vi "FPGA Image Acquisition (FPGA).vi"() -> ()   [LabVIEW 2013]
doc: "This is the FPGA VI for the 10-Tap 8-Bit Camera with DRAM example. This example demonstrates how to acquire images from a 10-tap, 8-bit, extended configuration, Camera Link camera and transfer the images to the host. This example supports area scan and line scan cameras for both continuous and finite acquisitions.\n\nThis example also demonstrates the use of DRAM as a frame buffer for very high speed acquisitions. Data packing and flow-control are also employed to maximize use of the available DRAM and FIFOs in terms of both memory space and performance.\n\nAdditionally, the example demonstrates the serial server, which allows third-party camera configuration utilities to communicate with the camera using the Camera Link serial interface while this VI is running."
uses:
  Common/CL Signal Mapping.ctl
  Common/CL Configuration.ctl
  <vilib>/Platform/TimedLoop/XDataNode/timing_clust.ctl
  <vilib>/Platform/TimedLoop/XDataNode/nitl_modes.ctl
  <vilib>/Platform/TimedLoop/XDataNode/wakeup.ctl
  <vilib>/rvi/Emulation/niFpgaSctlEmulationGetInTimedLoop.vi
  <vilib>/rvi/Emulation/niFpgaEmulationReportErrorSimple.vi
  <vilib>/rvi/eio/common/nirviEmuTemplateMethod_errors.vi
  <vilib>/rvi/Emulation/niFpgaGetClockAttributes.vi
  <vilib>/rvi/Emulation/niFpgaCriticalErrorInLSC.vi
  Common/CL Data to Pixels/10 Tap 8-Bit.vi
  <vilib>/rvi/interface/RandomDataEmulation/nirviRandomDataFPGAFIFO.vi
  <vilib>/rvi/interface/RandomDataEmulation/niFpgaRandomDataHandleErrors.vi
  <vilib>/rvi/FIFO/Fifo_Resource/nirvififoEmulationWriteFpgaImpl.vi
  <vilib>/rvi/DataTransferAndStorage/Container/Common/niFpgaContainerGetUniqueNameForEmu.vi
  <vilib>/rvi/FIFO/Fifo_Resource/nirvififoEmulationGetNumberOfElementsToReadFpgaImpl.vi
  <vilib>/rvi/FIFO/Fifo_Resource/nirvififoEmulationReadFpgaImpl.vi
  <vilib>/rvi/Emulation/niFpgaProcessEmulError.vi
  <vilib>/Platform/TimedLoop/XDataNode/XDataNode.xnode
  <vilib>/eio/EIONode/EIONode.xnode
  <vilib>/rvi/DataTransferAndStorage/Container/XNode/niFpgaContainer.xnode
  <vilib>/rvi/interface/RandomDataEmulation/nirviRandomDataFpgaReadWriteTemplate.vi
  <vilib>/rvi/FIFO/Fifo_Resource/nirvififoEmulationWrite.vi
  <vilib>/rvi/FIFO/Fifo_Resource/nirvififoEmulationGetNumberOfElementsToRead.vi
  <vilib>/rvi/FIFO/Fifo_Resource/nirvififoEmulationRead.vi
  <vilib>/Platform/TimedLoop/XDataNode/XDNodeRunTimeDep.lvlib
panel:
  in  "CL Config.Configuration":T1=enum."Full"
  in  "CL Config.Signal Mapping":T2=enum."Basler 10-tap"
  in  "CL Config.Line Scan":bool
  in  "CL Config.DVAL Active High":bool=TRUE
  in  "CL Config.LVAL Active High":bool=TRUE
  in  "CL Config.FVAL Active High":bool=TRUE
  in  "CL Config.Spare Active High":bool=TRUE
  in  "Acq Control.Line Scan Height":u32
  in  "Acq Control.Frames To Acq":u32
  in  "Acq Control.Acquire":bool
  in  "Acq Control.Cancel Acq":bool
  in  "Acq Control.Ignore DVAL":bool
  in  "Acq Control.Initialize":bool
  out "Acq Status.Acq In Progress":bool
  out "Acq Status.Clocks Per Line":u32
  out "Acq Status.Frames Acq'd":u32
  out "Acq Status.Lines Per Frame":u32
  out "Acq Status.DMA Write Timeout":bool
  out "Acq Status.Initialized":bool
  in  "UART.Baud Rate":u8
  in  "UART.Transmit":bool
  in  "UART.Tx Data":u8[](array[numeric])=[0, 0, 0, 0, 0, 0, 0, 0, 0, 0] format="%02x"
  in  "UART.Set Baud Rate":bool
  in  "UART.Byte Mode":bool=TRUE
  out "UART.Rx Ready":bool
  out "UART.Break Indicator":bool
  out "UART.Framing Error":bool
  out "UART.Overrun Error":bool
  out "UART.Tx Ready":bool
  out "UART.Rx Data":u8 format="%02x"
  in  "UART.Receive":bool
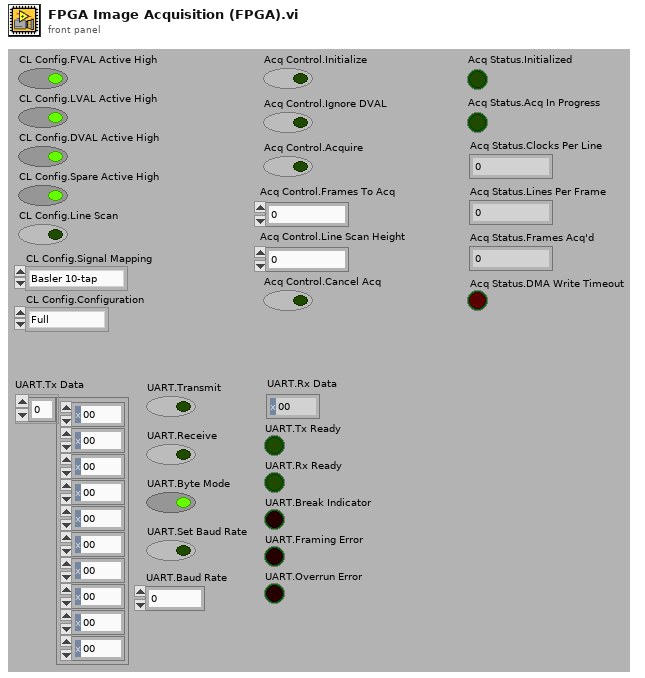
[diagram p1: front panel]
types:
  T1 = typedef "CL Configuration.ctl" = enum8{"Base", "Medium", "Full"}
  T2 = typedef "CL Signal Mapping.ctl" = enum8{"Standard", "Basler 10-tap", "Vosskühler 10-tap"}
  T3 = typedef "XDNodeRunTimeDep.lvlib/timing_clust.ctl" = cluster{"Expected End [f-1]":u64, "Actual End [f-1]":u64, "Finished Late? [f-1]":bool, "Expected End [i-1]":u64, "Actual End [i-1]":u64, "Finished Late? [i-1]":bool, "Expected Start [i]":u64, "Actual Start [i]":u64, "Expected Start [f]":u64, "Actual Start [f]":u64, "Source Name":string, "Structure Name":string, "Period":i64, "Deadline":i64, "Offset":i64, "Start":i64, "Priority":i32, "Timeout":i32, "Mode":T4, "Wakeup Reason":T5, "Error":errorcluster, "Source Type":string, "Secondary Source Type":string, "Global End Time":u64, "Global Start Time":u64, "Frame Duration":u64, "Iteration Duration":u64, "Assigned CPU":i32, "I/O Scan Engine Mode":u32}
  T4 = typedef "XDNodeRunTimeDep.lvlib/nitl_modes.ctl" = enum32{"No Change", "Process missed periods, maintain original phase", "Discard missed periods, maintain original phase", "Process missed periods, ignore original phase", "Discard missed periods, ignore original phase"}
  T5 = typedef "XDNodeRunTimeDep.lvlib/wakeup.ctl" = enum32{"Normal", "Aborted", "Asynchronous wakeup", "Timing source error", "Timed loop error", "Timeout"}
  T6 = cluster{"Enables Valid":bool, "Frame Valid":bool, "Line Valid":bool, "Data Valid":bool}
  T7 = cluster{"Pixel 0":u8, "Pixel 1":u8, "Pixel 2":u8, "Pixel 3":u8, "Pixel 4":u8, "Pixel 5":u8, "Pixel 6":u8, "Pixel 7":u8, "Pixel 8":u8, "Pixel 9":u8}
  T8 = cluster{"Tx Data":u8[], "Transmit":bool, "Receive":bool, "Byte Mode":bool, "Set Baud Rate":bool, "Baud Rate":u8}
  T9 = cluster{"Rx Data":u8, "Turn Off Transmit":bool, "Turn Off Receive":bool, "Turn Off Set Baud Rate":bool, "Tx Ready":bool, "Rx Ready":bool, "Break Indicator":bool, "Framing Error":bool, "Overrun Error":bool}
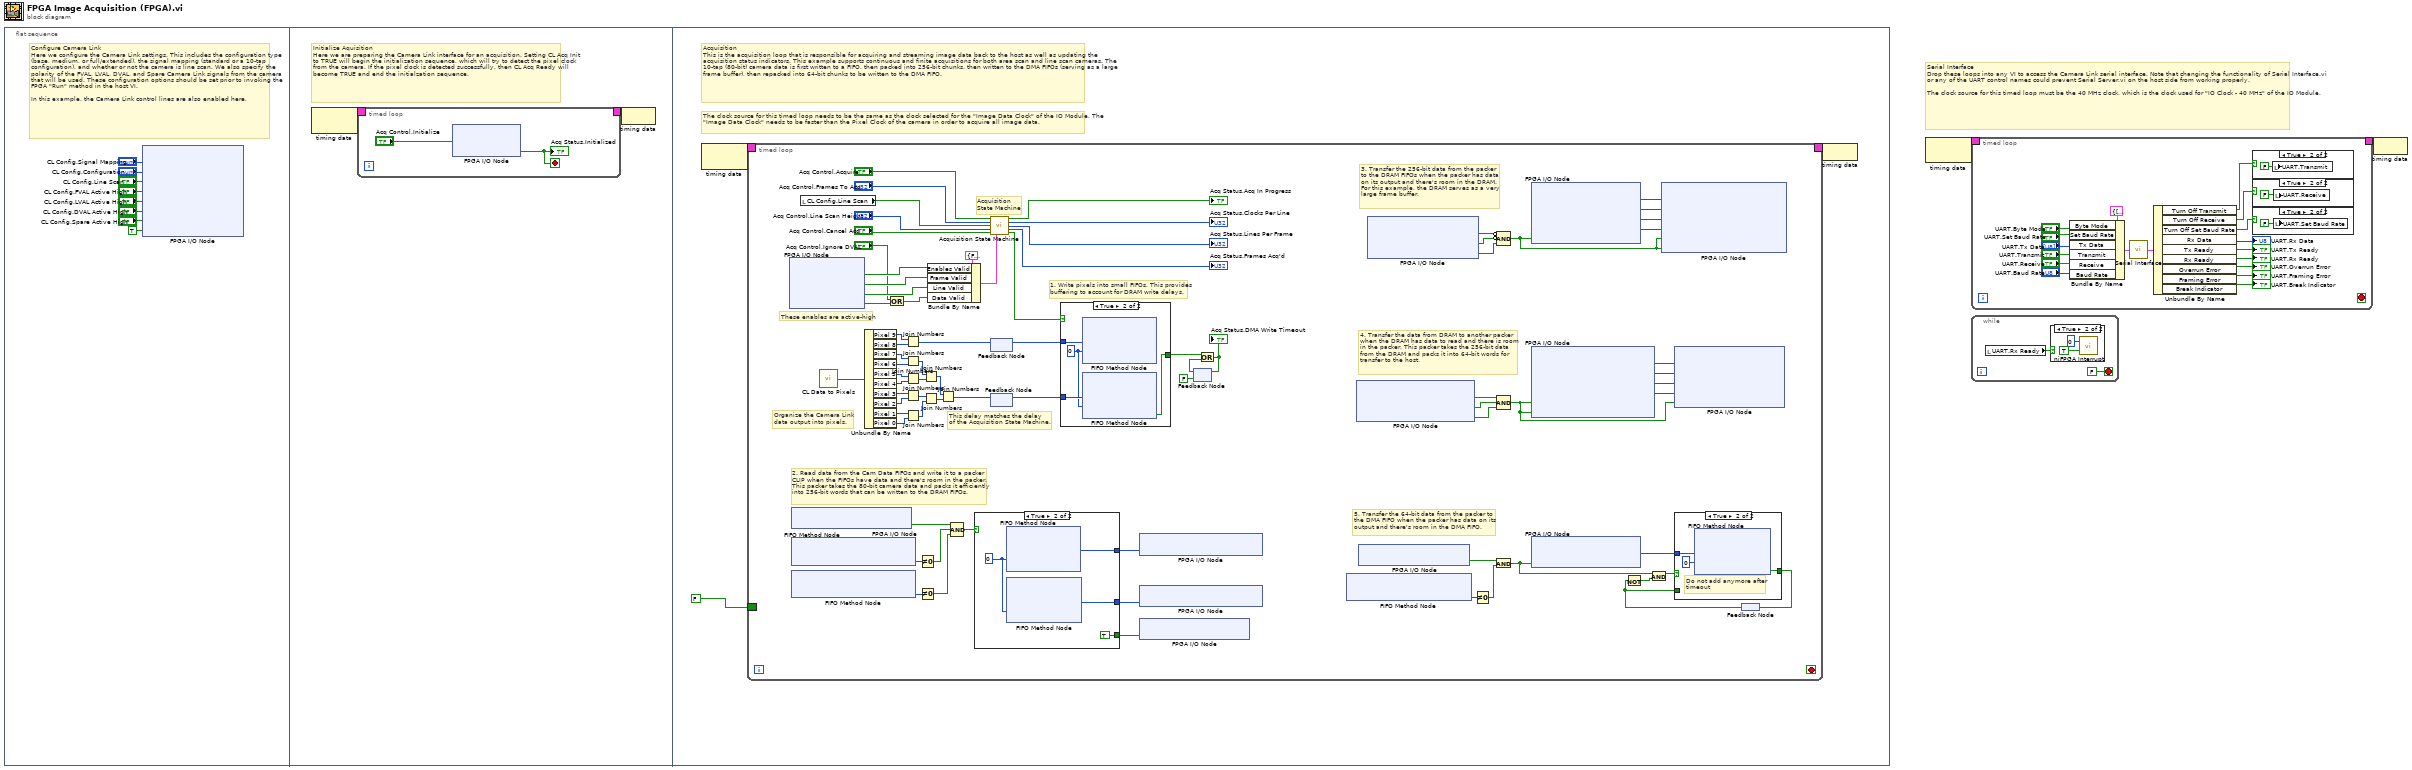
[diagram p0: block diagram]
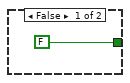
[diagram p8: hidden frame]
diagram:
  # "Serial Interface\nDrop these loops into any VI to access the Camera Link serial interface. Note that changing the functionality of Serial Interface.vi or any of the UART control names could prevent Serial Server.vi on the host side from working properly.\n\nThe clock source for this timed loop must be the 40 MHz clock, which is the clock used for \"IO Clock - 40 MHz\" of the IO Module."
  n1 = flat-sequence {
    frame #0 {
      # "Configure Camera Link\nHere we configure the Camera Link settings. This includes the configuration type (base, medium, or full/extended), the signal mapping (standard or a 10-tap configuration), and whether or not the camera is line scan. We also specify the polarity of the FVAL, LVAL, DVAL, and Spare Camera Link signals from the camera that will be used. These configuration options should be set prior to invoking the FPGA \"Run\" method in the host VI.\n\nIn this example, the Camera Link control lines are also enabled here."
      n2 = xnode "FPGA I/O Node"("CL Set Signal Mapping"="CL Config.Signal Mapping", "CL Set Configuration"="CL Config.Configuration", "CL Set Line Scan"="CL Config.Line Scan", "CL Set FVAL Active High"="CL Config.FVAL Active High", "CL Set LVAL Active High"="CL Config.LVAL Active High", "CL Set DVAL Active High"="CL Config.DVAL Active High", "CL Set Spare Active High"="CL Config.Spare Active High", "CL Control Enable"=TRUE ("IO Module\\CL Control Enable")) -> ()  [unwired: 8 in, 8 out]
    }
    frame #1 {
      # "Initialize Aquisition\nHere we are preparing the Camera Link interface for an acquisition. Setting CL Acq Init to TRUE will begin the initialization sequence, which will try to detect the pixel clock from the camera. If the pixel clock is detected successfully, then CL Acq Ready will become TRUE and end the initialzation sequence."
      n3 = node-c288() -> (w12:T3)  [unwired: 1 out]
      n4 = timed-loop {
        timing: w12 -> [_]
        timing-out: [_] -> w11
        stop <- w13 stop-if-true
        n5 = xnode "FPGA I/O Node"("CL Acq Init"="Acq Control.Initialize") -> ("CL Acq Ready"=w13:bool)  [unwired: 2 in, 2 out]
        "Acq Status.Initialized" <- w13
      }
      n6 = node-c288(w11) -> ()
    }
    frame #2 {
      # "The clock source for this timed loop needs to be the same as the clock selected for the \"Image Data Clock\" of the IO Module. The \"Image Data Clock\" needs to be faster than the Pixel Clock of the camera in order to acquire all image data."
      # "Acquisition\nThis is the acquisition loop that is responsible for acquiring and streaming image data back to the host as well as updating the acquisition status indicators. This example supports continuous and finite acquisitions for both area scan and line scan cameras. The 10-tap (80-bit) camera data is first written to a FIFO, then packed into 256-bit chunks, then written to the DMA FIFOs (serving as a large frame buffer), then repacked into 64-bit chunks to be written to the DMA FIFO."
      n7 = node-c288() -> (w21:T3)  [unwired: 1 in]
      n8 = timed-loop {
        timing: w21 -> [_]
        timing-out: [_] -> w20
        border: FALSE ("Timed Out?") -> [_]
        stop <- _ stop-if-true
        # "3. Transfer the 256-bit data from the packer\nto the DRAM FIFOs when the packer has data\non its output and there's room in the DRAM.\nFor this example, the DRAM serves as a very\nlarge frame buffer."
        # "5. Transfer the 64-bit data from the packer to\nthe DMA FIFO when the packer has data on its\noutput and there's room in the DMA FIFO."
        # "4. Transfer the data from DRAM to another packer\nwhen the DRAM has data to read and there is room\nin the packer. This packer takes the 256-bit data\nfrom the DRAM and packs it into 64-bit words for\ntransfer to the host."
        # "2. Read data from the Cam Data FIFOs and write it to a packer\nCLIP when the FIFOs have data and there's room in the packer.\nThis packer takes the 80-bit camera data and packs it efficiently\ninto 256-bit words that can be written to the DRAM FIFOs."
        # "1. Write pixels into small FIFOs. This provides\nbuffering to account for DRAM write delays."
        # "Organize the Camera Link\ndata output into pixels."
        # "These enables are active-high"
        # "This delay matches the delay\nof the Acquisition State Machine."
        # "Acquisition\nState Machine"
        n9 = xnode "FPGA I/O Node"() -> ("CL Output Valid"=w84:bool, "CL Frame Valid"=w83:bool, "CL Line Valid"=w82:bool, "CL Data Valid"=w79:bool)  [unwired: 4 in, 4 out]
        n10 = xnode "FPGA I/O Node"() -> ("Pack 80 to 256\\Ready For Write"=w27:bool)  [unwired: 1 in, 1 out]
        n11 = xnode ("FIFO Method Node")() -> ("Number of Elements to Read"=w55:u32)  [unwired: 1 in, 1 out]
        n12 = xnode ("FIFO Method Node")() -> ("Number of Elements to Read"=w54:u32)  [unwired: 1 in, 1 out]
        n13 = local read "CL Config.Line Scan"() -> (w76:bool)
        n14 = call-poly "CL Data to Pixels.vi"() -> ("Pixels"=w98:T7)  [unwired: 1 in]
        n15 = Unbundle By Name(w98) -> ("Pixel 9"=w74:u8, "Pixel 8"=w73:u8, "Pixel 7"=w72:u8, "Pixel 6"=w71:u8, "Pixel 5"=w70:u8, "Pixel 4"=w69:u8, "Pixel 3"=w68:u8, "Pixel 2"=w67:u8, "Pixel 1"=w66:u8, "Pixel 0"=w65:u8)
        n16 = Or(x="Acq Control.Ignore DVAL", y=w79) -> (x .or. y?=w78:bool)
        n17 = Join Numbers(hi=w74, lo=w73) -> ((hi.lo)=w60:u16)
        n18 = Join Numbers(hi=w72, lo=w71) -> ((hi.lo)=w63:u16)
        n19 = Join Numbers(hi=w70, lo=w69) -> ((hi.lo)=w62:u16)
        n20 = Join Numbers(hi=w68, lo=w67) -> ((hi.lo)=w61:u16)
        n21 = Join Numbers(hi=w66, lo=w65) -> ((hi.lo)=w64:u16)
        n22 = Not Equal To 0?(x=w55) -> (x != 0?=w52:bool)
        n23 = Not Equal To 0?(x=w54) -> (x != 0?=w51:bool)
        n24 = Join Numbers(hi=w63, lo=w62) -> ((hi.lo)=w59:u32)
        n25 = Join Numbers(hi=w61, lo=w64) -> ((hi.lo)=w58:u32)
        n26 = Bundle By Name(cluster=T6 {"Enables Valid"=FALSE, "Frame Valid"=FALSE, "Line Valid"=FALSE, "Data Valid"=FALSE} ("Enables"), "Enables Valid"=w84, "Frame Valid"=w83, "Line Valid"=w82, "Data Valid"=w78) -> (w81:T6)
        n27 = Join Numbers(hi=w59, lo=w58) -> ((hi.lo)=w57:u64)
        n28 = Compound Arithmetic op=AND(w27, w52, w51) -> (w53:bool)
        n29 = case shown="True" w53 {
          tunnel: [_ w106] -> w30
          tunnel: [_ w105] -> w29
          tunnel: [_ TRUE] -> w28
          frame False {
          }
          frame True {
            w104 = 0 ("Timeout")
            n30 = xnode ("FIFO Method Node")("Timeout"=w104) -> ("Element"=w106:u16)  [unwired: 1 in, 2 out]
            n31 = xnode ("FIFO Method Node")("Timeout"=w104) -> ("Element"=w105:u64)  [unwired: 1 in, 2 out]
          }
        }
        n32 = call "Acquisition State Machine.vi"("Acquire"="Acq Control.Acquire", "Frames to Acquire"="Acq Control.Frames To Acq", "Line Scan"=w76, "Line Scan Height"="Acq Control.Line Scan Height", "Cancel Acq"="Acq Control.Cancel Acq", "Enables"=w81) -> ("Acq In Progress"=→"Acq Status.Acq In Progress":bool, "Num Clocks Per Line"=→"Acq Status.Clocks Per Line":u32, "Num Lines Per Frame"=→"Acq Status.Lines Per Frame":u32, "Num Frames Acq'd"=→"Acq Status.Frames Acq'd":u32, "Capture Cycle"=w96:bool)  [unwired: 4 in, 1 out]
        n33 = feedback #1() -> (w56:u16)  [unwired: 1 in]
        n34 = feedback-in #1(w60) -> ()
        n35 = feedback-in #2(w57) -> ()
        n36 = feedback #2() -> (w97:u64)  [unwired: 1 in]
        n37 = case shown="True" w96 {
          tunnel: [FALSE ("Timed Out?") w110] -> w94
          tunnel: w97 -> [_ w111]
          tunnel: w56 -> [_ w109]
          frame False {
          }
          frame True {
            w108 = 0 ("Timeout")
            n38 = xnode ("FIFO Method Node")("Element"=w109, "Timeout"=w108) -> ()  [unwired: 1 in, 2 out]
            n39 = xnode ("FIFO Method Node")("Element"=w111, "Timeout"=w108) -> ("Timed Out?"=w110:bool)  [unwired: 1 in, 1 out]
          }
        }
        n40 = xnode "FPGA I/O Node"("Pack 80 to 256\\Data In Upper 16"=w30) -> ()  [unwired: 1 in, 1 out]
        n41 = xnode "FPGA I/O Node"("Pack 80 to 256\\Data In Lower 64"=w29) -> ()  [unwired: 1 in, 1 out]
        n42 = xnode "FPGA I/O Node"("Pack 80 to 256\\Write Enable"=w28) -> ()  [unwired: 1 in, 1 out]
        n43 = feedback #3(FALSE) -> (w93:bool)
        n44 = Or(x=w94, y=w93) -> (x .or. y?=w92:bool)
        "Acq Status.DMA Write Timeout" <- w92
        n45 = feedback-in #3(w92) -> ()
        n46 = xnode ("FIFO Method Node")() -> ("Number of Elements to Write"=w40:u32)  [unwired: 1 in, 1 out]
        n47 = xnode "FPGA I/O Node"() -> ("DRAM Bank 1\\Data_Available"=w50:bool, "DRAM Bank 0\\Data_Available"=w48:bool, "Pack 256 to 64\\Ready for Write"=w49:bool)  [unwired: 3 in, 3 out]
        n48 = xnode "FPGA I/O Node"() -> ("Pack 256 to 64\\Output Valid"=w42:bool)  [unwired: 1 in, 1 out]
        n49 = xnode "FPGA I/O Node"() -> ("DRAM Bank 1\\Full"=w34:bool, "DRAM Bank 0\\Full"=w35:bool, "Pack 80 to 256\\Output Valid"=w26:bool)  [unwired: 3 in, 3 out]
        n50 = Not Equal To 0?(x=w40) -> (x != 0?=w41:bool)
        n51 = And(x=w42, y=w41) -> (x .and. y?=w31:bool)
        n52 = Compound Arithmetic op=AND(invert w34, invert w35, w26) -> (w33:bool)
        n53 = Compound Arithmetic op=AND(w50, w48, w49) -> (w32:bool)
        n54 = xnode "FPGA I/O Node"("Pack 80 to 256\\Read Enable"=w33) -> ("Pack 80 to 256\\Data Out 3"=w36:u64, "Pack 80 to 256\\Data Out 2"=w37:u64, "Pack 80 to 256\\Data Out 1"=w39:u64, "Pack 80 to 256\\Data Out 0"=w38:u64)  [unwired: 5 in, 5 out]
        n55 = xnode "FPGA I/O Node"("DRAM Bank 1\\Read"=w32, "DRAM Bank 0\\Read"=w32) -> ("DRAM Bank 1\\Read_Data_Upper"=w46:u64, "DRAM Bank 1\\Read_Data_Lower"=w45:u64, "DRAM Bank 0\\Read_Data_Upper"=w44:u64, "DRAM Bank 0\\Read_Data_Lower"=w43:u64)  [unwired: 6 in, 6 out]
        n56 = xnode "FPGA I/O Node"("Pack 256 to 64\\Read Enable"=w31) -> ("Pack 256 to 64\\Data Out 64"=w47:u64)  [unwired: 2 in, 2 out]
        n57 = xnode "FPGA I/O Node"("DRAM Bank 1\\Write_Data_Upper"=w36, "DRAM Bank 1\\Write_Data_Lower"=w37, "DRAM Bank 0\\Write_Data_Upper"=w39, "DRAM Bank 0\\Write_Data_Lower"=w38, "DRAM Bank 1\\Write"=w33, "DRAM Bank 0\\Write"=w33) -> ()  [unwired: 6 in, 6 out]
        n58 = xnode "FPGA I/O Node"("Pack 256 to 64\\Data In 3"=w46, "Pack 256 to 64\\Data In 2"=w45, "Pack 256 to 64\\Data In 1"=w44, "Pack 256 to 64\\Data In 0"=w43, "Pack 256 to 64\\Write Enable"=w32) -> ()  [unwired: 5 in, 5 out]
        n59 = feedback #4() -> (w22:bool)
        n60 = Not(x=w22) -> (.not. x?=w23:bool)
        n61 = And(x=w31, y=w23) -> (x .and. y?=w25:bool)
        n62 = case shown="True" w25 {
          tunnel: w47 -> [_ w102]
          tunnel: [w99 w100] -> w24
          tunnel: w22 -> [w99 _]
          frame False {
          }
          frame True {
            # "Do not add anymore after\ntimeout"
            n63 = xnode ("FIFO Method Node")("Element"=w102, "Timeout"=0) -> ("Timed Out?"=w100:bool)  [unwired: 1 in, 1 out]
          }
        }
        n64 = feedback-in #4(w24) -> ()
      }
      n65 = node-c288(w20) -> ()
    }
  }
  n66 = node-c288() -> (w2:T3)  [unwired: 1 out]
  n67 = timed-loop {
    timing: w2 -> [_]
    timing-out: [_] -> w1
    stop <- _ stop-if-true
    n68 = Bundle By Name(cluster=T8 {"Tx Data"=[0, 0, 0, 0, 0, 0, 0, 0, 0, 0], "Transmit"=FALSE, "Receive"=FALSE, "Byte Mode"=TRUE, "Set Baud Rate"=FALSE, "Baud Rate"=0} ("UART Inputs"), "Byte Mode"="UART.Byte Mode", "Set Baud Rate"="UART.Set Baud Rate", "Tx Data"="UART.Tx Data", "Transmit"="UART.Transmit", "Receive"="UART.Receive", "Baud Rate"="UART.Baud Rate") -> (w116:T8)
    n69 = call "Serial Interface.vi"("UART Inputs"=w116) -> ("UART Outputs"=w128:T9)
    n70 = Unbundle By Name(w128) -> ("Turn Off Transmit"=w121:bool, "Turn Off Receive"=w122:bool, "Turn Off Set Baud Rate"=w118:bool, "Rx Data"=→"UART.Rx Data":u8, "Tx Ready"=→"UART.Tx Ready":bool, "Rx Ready"=→"UART.Rx Ready":bool, "Overrun Error"=→"UART.Overrun Error":bool, "Framing Error"=→"UART.Framing Error":bool, "Break Indicator"=→"UART.Break Indicator":bool)
    n71 = case shown="True" w121 {
      frame False {
      }
      frame True {
        n72 = local write "UART.Transmit"(FALSE ("UART.Transmit")) -> ()
      }
    }
    n73 = case shown="True" w122 {
      frame False {
      }
      frame True {
        n74 = local write "UART.Receive"(FALSE ("UART.Receive")) -> ()
      }
    }
    n75 = case shown="True" w118 {
      frame False {
      }
      frame True {
        n76 = local write "UART.Set Baud Rate"(FALSE ("UART.Receive")) -> ()
      }
    }
  }
  n77 = while {
    stop <- FALSE stop-if-true
    n78 = local read "UART.Rx Ready"() -> (w140:bool)
    n79 = case shown="True" w140 {
      frame False {
      }
      frame True {
        n80 = call <vilib>:"niFPGA Interrupt.vi"("Wait Until Cleared (F)"=TRUE ("Wait Until Cleared"), "IRQ Number (0)"=u8 0 ("IRQ Number")) -> ()  [unwired: 1 in]
      }
    }
  }
  n81 = node-c288(w1) -> ()
